vi "CallBack_SizeChanged.vi"(4 "reference in":refnum<class "LcPictureBox.lvclass">, 5 "Event Data":cluster{"sender":refnum<k24>, "e":refnum<k24>}, 6 "Control Ref":refnum<k24>, 7 "Event Common Data":T1) -> ()   [LabVIEW 2020, in "LcPictureBox.lvclass"]
uses:
  LcPictureBox.lvclass
  System.Windows.Forms
panel:
  out "Height":i32
  out "Width":i32
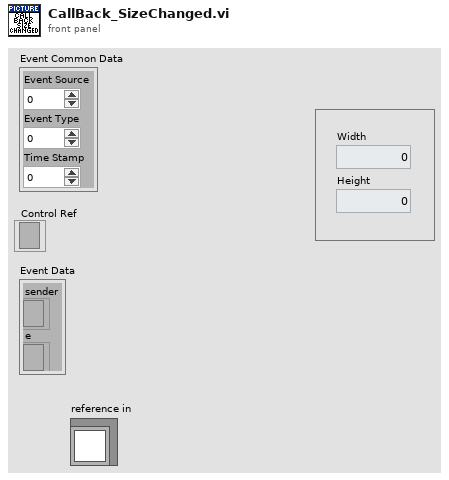
[diagram p1: front panel]
types:
  T1 = cluster{"Event Source":i32, "Event Type":u32, "Time Stamp":u32}
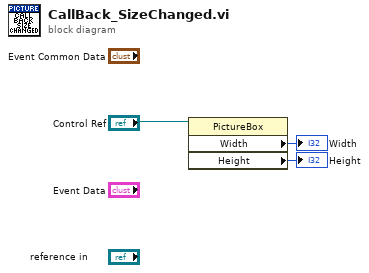
[diagram p0: block diagram]
diagram:
  n1 = property on="Property Node" class="PictureBox"(reference="Control Ref") -> ("Width"=→"Width":i32, "Height"=→"Height":i32)  [unwired: 1 in, 2 out]
